vi "dfd_FXP Lattice One Multiplier Section.vi"(4 "FXPOPs":T4[](array[typedef]) {"source" items=["Coef a/k"=0, "Coef b/v"=7, "Input"=1, "Output"=2, "Multiplicand"=3, "Product"=4, "Sum"=5, "Delay"=6, "Gain"=8]}, 5 "filtering statistics in":T3(array[cluster]) {"statistics information"."min value" format="%.2f"; "statistics information"."max value" format="%.2f"; "Quantizer Source" items=["Coefficients a/k"=0, "Coefficients b/v"=7, "Input"=1, "Output"=2, "Multiplicand"=3, "Product"=4, "Sum"=5, "Delay"=6]}, 6 "k(m)":T6={"value"=0, "wl"=0, "iwl"=0, "Signed"=TRUE} {"value" format="%.0x"}, 7 "w(m-1)":T6={"value"=0, "wl"=0, "iwl"=0, "Signed"=TRUE} {"value" format="%.0x"}, 8 "x(m)":T6={"value"=0, "wl"=0, "iwl"=0, "Signed"=TRUE} {"value" format="%.0x"}) -> (0 "filtering statistics out":T3(array[cluster]) {"statistics information"."min value" format="%.2f"; "statistics information"."max value" format="%.2f"; "Quantizer Source" items=["Coefficients a/k"=0, "Coefficients b/v"=7, "Input"=1, "Output"=2, "Multiplicand"=3, "Product"=4, "Sum"=5, "Delay"=6]}, 2 "w(m)":T6={"value"=0, "wl"=0, "iwl"=0, "Signed"=TRUE} {"value" format="%.0x"}, 3 "x(m-1)":T6={"value"=0, "wl"=0, "iwl"=0, "Signed"=TRUE} {"value" format="%.0x"})   [LabVIEW 2017, in "NI_DigFilter_FXP.lvlib"]
uses:
  <vilib>/addons/Digital Filter Design/NI_DigFilter_FXP.lvlib
  <vilib>/addons/Digital Filter Design/_Objects.llb/dfd_DFXP Data Type (scaler).ctl
  <vilib>/addons/Digital Filter Design/_Objects.llb/dfd_DFXP Operation Parameter.ctl
  <vilib>/addons/Digital Filter Design/_Objects.llb/dfd_Internal Quantization Srcs.ctl
  <vilib>/addons/Digital Filter Design/_Objects.llb/DFD Quantization Sources.ctl
  <vilib>/addons/Digital Filter Design/_Objects.llb/DFD FXP Statistics Data.ctl
  <vilib>/addons/Digital Filter Design/NI_DigFilterLicensed.lvlib
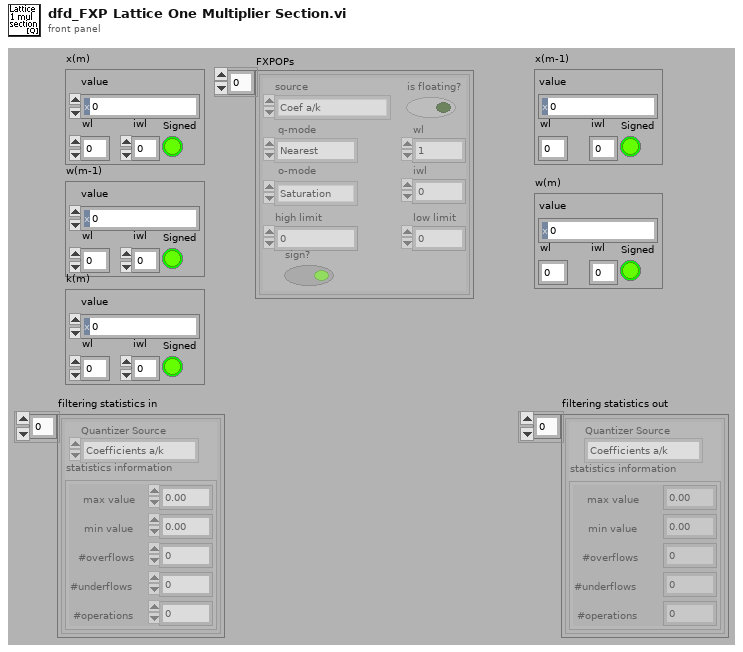
[diagram p1: front panel]
types:
  T1 = typedef "NI_DigFilterLicensed.lvlib/DFD Quantization Sources.ctl" = u16
  T2 = typedef "NI_DigFilterLicensed.lvlib/DFD FXP Statistics Data.ctl" = cluster{"max value":ext, "min value":ext, "#overflows":i32, "#underflows":i32, "#operations":i32}
  T3 = cluster{"Quantizer Source":T1, "statistics information":T2}[]
  T4 = typedef "dfd_DFXP Operation Parameter.ctl" = cluster{"source":T5, "is floating?":bool, "o-mode":enum16{"Saturation", "Wrap"}, "q-mode":enum16{"Nearest", "Truncation"}, "wl":i16, "high limit":i64, "low limit":i64, "iwl":i16, "sign?":bool}
  T5 = typedef "NI_DigFilterLicensed.lvlib/dfd_Internal Quantization Srcs.ctl" = u16
  T6 = typedef "dfd_DFXP Data Type (scaler).ctl" = cluster{"value":i64, "wl":i16, "iwl":i16, "Signed":bool}
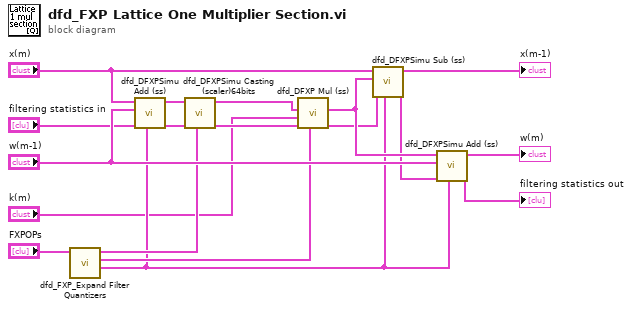
[diagram p0: block diagram]
diagram:
  n1 = call <vilib>:"dfd_FXP_Expand Filter Quantizers.vi"("FXPOPs"="FXPOPs") -> ("Sum"=w4:T4, "Product"=w6:T4, "Multiplicand"=w7:T4)  [unwired: 8 out]
  n2 = call <vilib>:"dfd_DFXPSimu Add (ss).vi"("op params"=w4, "filtering statistics in"="filtering statistics in", "value in 2"="w(m-1)", "value in 1"="x(m)") -> ("filtering statistics out"=w10:T3, "value out"=w13:T6)  [unwired: 1 in, 5 out]
  n3 = call <vilib>:"dfd_DFXPSimu Casting (scaler)64bits.vi"("op params"=w7, "filtering statistics in"=w10, "Value in"=w13) -> ("filtering statistics out"=w9:T3, "Value out"=w1:T6)  [unwired: 2 in, 5 out]
  n4 = call <vilib>:"dfd_DFXP Mul (ss).vi"("op params"=w6, "filtering statistics in"=w9, "Value in 2"="k(m)", "Value in"=w1) -> ("filtering statistics out"=w3:T3, "Value out"=w14:T6)  [unwired: 6 out]
  n5 = call <vilib>:"dfd_DFXPSimu Sub (ss).vi"("op params"=w4, "filtering statistics in"=w3, "value in 2"=w14, "value in 1"="x(m)") -> ("filtering statistics out"=w5:T3, "value out"=→"x(m-1)":T6)  [unwired: 1 in, 5 out]
  n6 = call <vilib>:"dfd_DFXPSimu Add (ss).vi"("op params"=w4, "filtering statistics in"=w5, "value in 2"="w(m-1)", "value in 1"=w14) -> ("filtering statistics out"=→"filtering statistics out":T3, "value out"=→"w(m)":T6)  [unwired: 1 in, 5 out]
